vi "waveform autocorrelation.vi"(8 "error in (no error)":errorcluster, 11 "signal in":waveform(dbl)={"t0"=timestamp(0 s since 1904-01-01), "dt"=0.0, "Y"=[]}) -> (0 "error out":errorcluster, 3 "convolved signal":waveform(dbl))   [LabVIEW 2020, in "NI_MAPro.lvlib"]
uses:
  NI_MAPro.lvlib
  NI_AALPro.lvlib
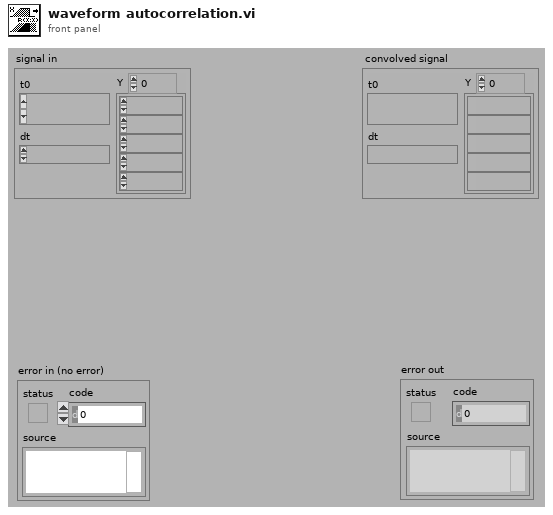
[diagram p1: front panel]
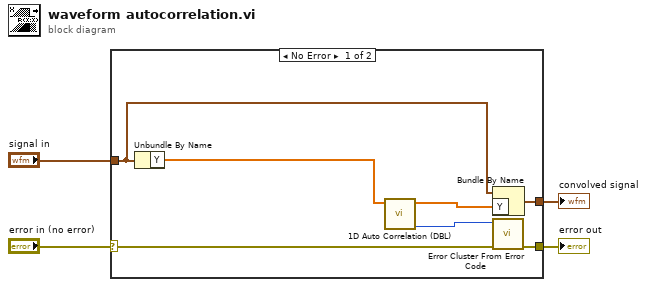
[diagram p0: block diagram]
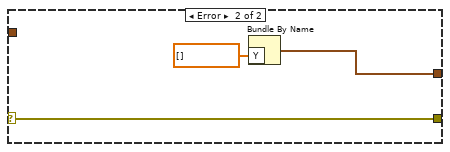
[diagram p2: hidden frame]
diagram:
  n1 = case shown="No Error" "error in (no error)" {
    selector: "error in (no error)" -> [w8 w14]
    tunnel: "signal in" -> [w6 _]
    tunnel: [w5 w13] -> w3
    tunnel: [w9 w14] -> w1
    frame No Error {
      n2 = Unbundle By Name(w6) -> ("Y"=w11:dbl[])
      n3 = call "1D Auto Correlation (DBL).vi"("X"=w11) -> ("error"=w10:i32, "Rxx"=w7:dbl[])  [unwired: 9 in]
      n4 = Bundle By Name(cluster=w6, "Y"=w7) -> (w5:waveform(dbl))
      n5 = call "Error Cluster From Error Code.vi"("error in (no error)"=w8, "error code (0)"=w10) -> ("error out"=w9:errorcluster)  [unwired: 7 in]
    }
    frame Error {
      n6 = Bundle By Name("Y"=dbl[] []) -> (w13:waveform(dbl))  [unwired: 1 in]
    }
  }
  "convolved signal" <- w3
  "error out" <- w1
